vi "ConfigPhases.vi"(8 "error in (no error)":errorcluster, 11 "ChromaAcLoad in":refnum<class "ChromaAcLoad.lvclass">) -> (0 "error out":errorcluster, 3 "ChromaAcLoad out":refnum<class "ChromaAcLoad.lvclass">)   [LabVIEW 2018, in "AcPwrPlugins.lvlib" / "ChromaAcLoad.lvclass"]
uses:
  ChromaAcLoad.lvclass
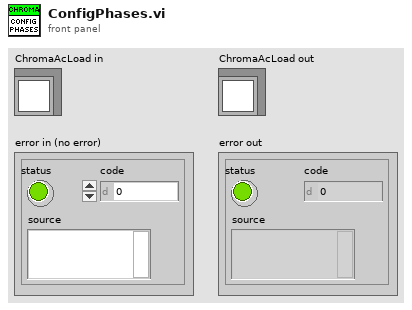
[diagram p1: front panel]
types:
  T1 = typedef "AcPwrPlugins.lvlib/ChromaAcLoad.lvclass/DeviceProperties.ctl" = cluster{"Frequency (Hz)":dbl, "Phases":cluster{"Handle":string, "Name":string, "Phase Select":i32, "option string ":string, "id query (Yes)":bool, "reset device (Yes)":bool, "LC":cluster{"C (uF)":i32, "L (uH)":i32, "RS (Ohm)":dbl, "RL (Ohm)":dbl}, "Load Current (A/Arms)":dbl, "Load Voltage (V/Vrms)":dbl, "Load Power (W)":dbl, "Load Resistance (Ohms)":dbl, "Load Current Peak (A)":dbl, "Load Current Limit (A/Arms)":dbl, "Slew Rate":cluster{"Rise Slew Rate (Units/S)":i32, "Fall Slew Rate (Units/S)":i32}, "Load Short Circuited":bool, "Line Synchronization":bool, "Priority":enum16{"CF Only", "PF Only", "Both (CF)", "Both (PF)"}, "Crest Factor":dbl, "Power Factor":dbl, "Connected":bool, "Voltage Range (V)":dbl[], "Timing":cluster{"TimingOn":enum16{""}, "Hours":u32, "Minutes":u32, "Seconds":dbl, "CutoffVoltage":dbl}}[], "Configuration Mode":enum16{"Constant Voltage (DC)", "Constant Power (DC)", "Constant Power (AC)", "Constant Current (DC)", "Constant Current (AC)", "Constant Resistance (DC)", "Constant Resistance (AC)", "Rectified Mode (DC)", "Inrush (AC)", "RLC CP (AC)", "RLC (AC)"}}[]
  T2 = cluster{"Handle":string, "Name":string, "Phase Select":i32, "option string ":string, "id query (Yes)":bool, "reset device (Yes)":bool, "LC":cluster{"C (uF)":i32, "L (uH)":i32, "RS (Ohm)":dbl, "RL (Ohm)":dbl}, "Load Current (A/Arms)":dbl, "Load Voltage (V/Vrms)":dbl, "Load Power (W)":dbl, "Load Resistance (Ohms)":dbl, "Load Current Peak (A)":dbl, "Load Current Limit (A/Arms)":dbl, "Slew Rate":cluster{"Rise Slew Rate (Units/S)":i32, "Fall Slew Rate (Units/S)":i32}, "Load Short Circuited":bool, "Line Synchronization":bool, "Priority":enum16{"CF Only", "PF Only", "Both (CF)", "Both (PF)"}, "Crest Factor":dbl, "Power Factor":dbl, "Connected":bool, "Voltage Range (V)":dbl[], "Timing":cluster{"TimingOn":enum16{""}, "Hours":u32, "Minutes":u32, "Seconds":dbl, "CutoffVoltage":dbl}}[]
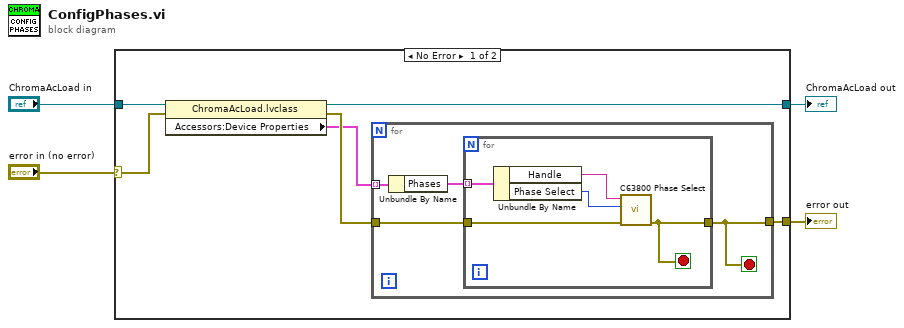
[diagram p0: block diagram]
diagram:
  n1 = case shown="No Error" "error in (no error)" {
    selector: "error in (no error)" -> [w9 w21]
    tunnel: "ChromaAcLoad in" -> [w10 w20]
    tunnel: [w8 w20] -> w2
    tunnel: [w5 w21] -> w1
    frame No Error {
      n2 = property class="ChromaAcLoad.lvclass"(reference=w10, error in=w9) -> (reference out=w8:refnum<class "ChromaAcLoad.lvclass">, error out=w7:errorcluster, "Accessors:Device Properties"=w6:T1)
      n3 = for {
        tunnel: w7 -> [w12]
        tunnel: w6 -> [w14] mode=indexing
        tunnel: [w11] -> w5
        stop <- w11 stop-if-true
        n4 = Unbundle By Name(w14) -> ("Phases"=w13:T2)
        n5 = for {
          tunnel: w13 -> [w17] mode=indexing
          tunnel: w12 -> [w19]
          tunnel: [w18] -> w11
          stop <- w18 stop-if-true
          n6 = Unbundle By Name(w17) -> ("Handle"=w16:string, "Phase Select"=w15:i32)
          n7 = call <instrlib>:"C63800 Phase Select.vi"("error in (no error)"=w19, "Phase Select"=w15, "Instrument Handle"=w16) -> ("error out"=w18:errorcluster)  [unwired: 7 in, 1 out]
        }
      }
    }
    frame Error {
    }
  }
  "error out" <- w1
  "ChromaAcLoad out" <- w2
